vi "Build Export Data File Path.vi"(9 "Meas name":string="ACMultiChannelMeasurement", 11 "Plugin name":string="DataConverter") -> (3 "Export data file path":path)   [LabVIEW 2021]
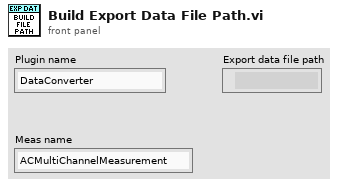
[diagram p1: front panel]
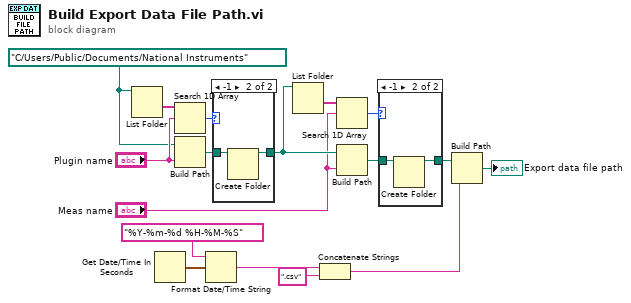
[diagram p0: block diagram]
diagram:
  w2 = path "C:/Users/Public/Documents/National Instruments" ("base path")
  n1 = List Folder(path=w2) -> (folder names=w16:string[])  [unwired: 3 in, 3 out]
  n2 = Get Date/Time In Seconds() -> (seconds since 1Jan1904=w7:timestamp)
  n3 = Search 1D Array(1D array=w16, element="Plugin name") -> (index of element=w14:i32)  [unwired: 1 in]
  n4 = Build Path(base path=w2, name or relative path="Plugin name") -> (appended path=w17:path)
  n5 = Format Date/Time String(time format string (%c)="%Y-%m-%d %H-%M-%S", seconds (now)=w7) -> (date/time string=w6:string)  [unwired: 1 in]
  n6 = case shown="-1" w14 {
    tunnel: w17 -> [w18 w20]
    tunnel: [w18 w19] -> w11
    frame Default {
    }
    frame -1 {
      n7 = Create Folder(path (use dialog)=w20) -> (created path=w19:path)  [unwired: 2 in, 2 out]
    }
  }
  n8 = List Folder(path=w11) -> (folder names=w13:string[])  [unwired: 3 in, 3 out]
  n9 = Concatenate Strings(w6, ".csv" ("string")) -> (w3:string)
  n10 = Search 1D Array(1D array=w13, element="Meas name") -> (index of element=w12:i32)  [unwired: 1 in]
  n11 = Build Path(base path=w11, name or relative path="Meas name") -> (appended path=w9:path)
  n12 = case shown="-1" w12 {
    tunnel: w9 -> [w21 w23]
    tunnel: [w21 w22] -> w4
    frame Default {
    }
    frame -1 {
      n13 = Create Folder(path (use dialog)=w23) -> (created path=w22:path)  [unwired: 2 in, 2 out]
    }
  }
  n14 = Build Path(base path=w4, name or relative path=w3) -> (appended path=→"Export data file path":path)
